vi "Elevator Choose Height.vi"(10 "Encoder Height":dbl, 11 "Elevator Settings Cluster":T1={"Ground Height"=0.0, "Switch Height"=0.0, "Scale High Height "=0.0, "Scale Low Height"=0.0, "Elevator PID Gains"={"proportional gain (Kc)"=1.0, "integral time (Ti, min)"=0.01, "derivative time (Td, min)"=0.0}, "High Output"=0.0, "Low Output"=0.0, "Elevator Tolerance"=0.0, "Reset Encoders"=FALSE} {"Elevator PID Gains"."derivative time (Td, min)" format="%.3f"; "Elevator PID Gains"."integral time (Ti, min)" format="%.3f"; "Elevator PID Gains"."proportional gain (Kc)" format="%.3f"}) -> (2 "Down":T3, 3 "Up":T3)   [LabVIEW 2017]
uses:
  Common Code/Elevator State.ctl
  Common Code/Elevator Settings Cluster.ctl
  Common Code/PID Gains.ctl
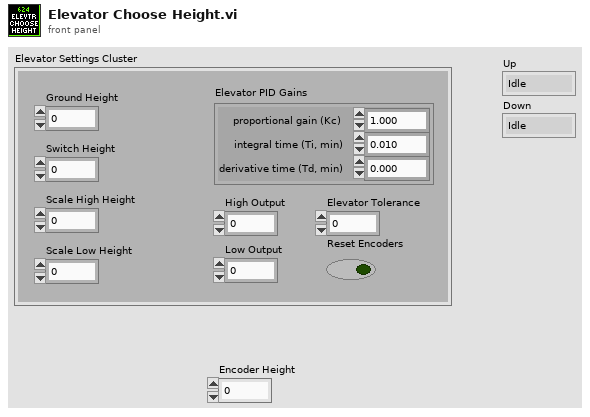
[diagram p1: front panel]
types:
  T1 = typedef "Elevator Settings Cluster.ctl" = cluster{"Ground Height":dbl, "Switch Height":dbl, "Scale High Height ":dbl, "Scale Low Height":dbl, "Elevator PID Gains":T2, "High Output":dbl, "Low Output":dbl, "Elevator Tolerance":dbl, "Reset Encoders":bool}
  T2 = typedef "PID Gains.ctl" = cluster{"proportional gain (Kc)":dbl, "integral time (Ti, min)":dbl, "derivative time (Td, min)":dbl}
  T3 = typedef "Elevator State.ctl" = enum16{"Idle", "Ground", "Scale High", "Scale Low", "Switch"}
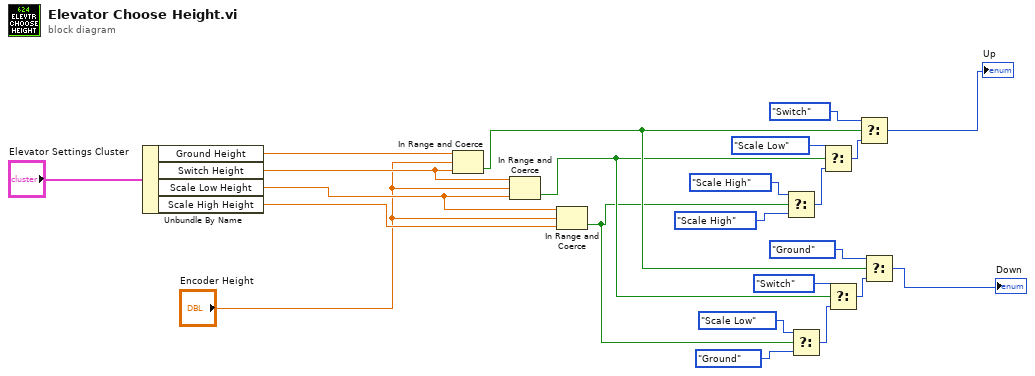
[diagram p0: block diagram]
diagram:
  n1 = Unbundle By Name("Elevator Settings Cluster") -> ("Ground Height"=w22:dbl, "Switch Height"=w21:dbl, "Scale Low Height"=w20:dbl, "Scale High Height"=w19:dbl)
  n2 = In Range and Coerce(upper limit=w22, x="Encoder Height", lower limit=w21) -> (In Range?=w3:bool)  [unwired: 1 out]
  n3 = In Range and Coerce(upper limit=w21, x="Encoder Height", lower limit=w20) -> (In Range?=w2:bool)  [unwired: 1 out]
  n4 = In Range and Coerce(upper limit=w20, x="Encoder Height", lower limit=w19) -> (In Range?=w1:bool)  [unwired: 1 out]
  n5 = Select(t=Elevator_State."Scale High" ("Up"), s=w1, f=Elevator_State."Scale High") -> (s? t:f=w13:T3)
  n6 = Select(t=Elevator_State."Scale Low" ("Up"), s=w1, f=Elevator_State."Ground") -> (s? t:f=w8:T3)
  n7 = Select(t=Elevator_State."Scale Low" ("Up"), s=w2, f=w13) -> (s? t:f=w15:T3)
  n8 = Select(t=Elevator_State."Switch" ("Up"), s=w2, f=w8) -> (s? t:f=w6:T3)
  n9 = Select(t=Elevator_State."Switch" ("Up"), s=w3, f=w15) -> (s? t:f=→"Up":T3)
  n10 = Select(t=Elevator_State."Ground" ("Up"), s=w3, f=w6) -> (s? t:f=→"Down":T3)
